vi "Validate Buffer Settings.vi"(11 "Buffered Log Sink in":refnum<class "Buffered String Log Sink.lvclass">) -> (0 "error out":errorcluster)   [LabVIEW 2018, in "MVA Framework.lvlib" / "Buffered String Log Sink.lvclass"]
uses:
  Buffered String Log Sink.lvclass
  <vilib>/ErrorRing/Error Ring.xnode
  <vilib>/Utility/error.llb/Error Cluster From Error Code.vi
  Composed Log/Log Sink/Log Sink.lvclass
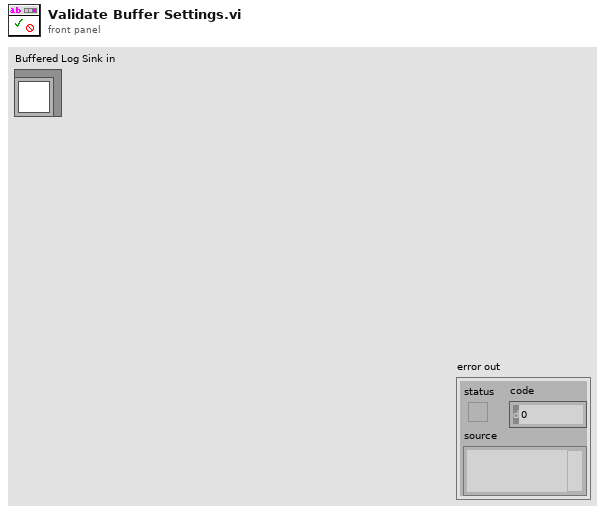
[diagram p1: front panel]
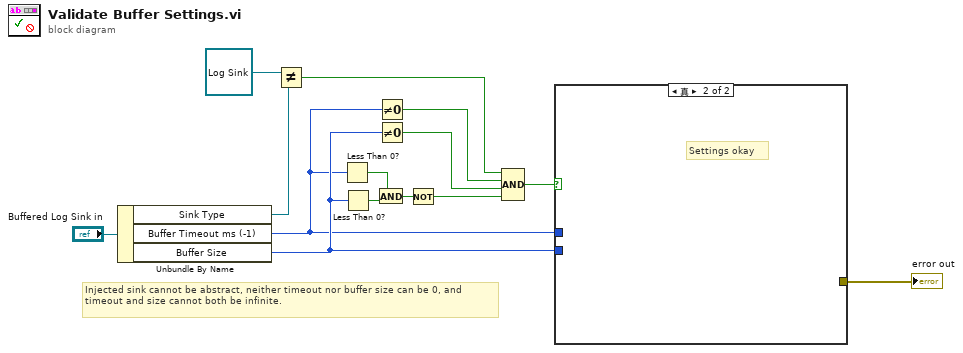
[diagram p0: block diagram]
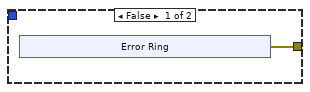
[diagram p2: hidden frame]
diagram:
  # "Injected sink cannot be abstract, neither timeout nor buffer size can be 0, and timeout and size cannot both be infinite."
  n1 = Unbundle By Name("Buffered Log Sink in") -> ("Sink Type"=w9:refnum<class "Log Sink.lvclass">, "Buffer Timeout ms (-1)"=w11:i32, "Buffer Size"=w12:i32)
  n2 = Not Equal?(x=refnum<class "Log Sink.lvclass"> refnum ("Sink"), y=w9) -> (x != y?=w2:bool)
  n3 = Less Than 0?(x=w11) -> (x < 0?=w7:bool)
  n4 = Less Than 0?(x=w12) -> (x < 0?=w8:bool)
  n5 = And(x=w7, y=w8) -> (x .and. y?=w6:bool)
  n6 = Not Equal To 0?(x=w11) -> (x != 0?=w3:bool)
  n7 = Not Equal To 0?(x=w12) -> (x != 0?=w4:bool)
  n8 = Not(x=w6) -> (.not. x?=w5:bool)
  n9 = Compound Arithmetic op=AND(w2, w3, w4, w5) -> (w1:bool)
  n10 = case shown="真" w1 {
    tunnel: w11 -> [_ _]
    tunnel: w12 -> [_ _]
    tunnel: [w15 _] -> w13
    frame False {
      n11 = xnode "Error Ring"() -> ("错误输出"=w15:errorcluster)
    }
    frame True {
      # "Settings okay"
    }
  }
  "error out" <- w13
